vi "Convert numbers to Quadruped String.vi"(11 "Body Movements":T1) -> (3 "String to Write to Quadruped":string)   [LabVIEW 2014]
panel:
  out "String to Write to Quadruped 2":string
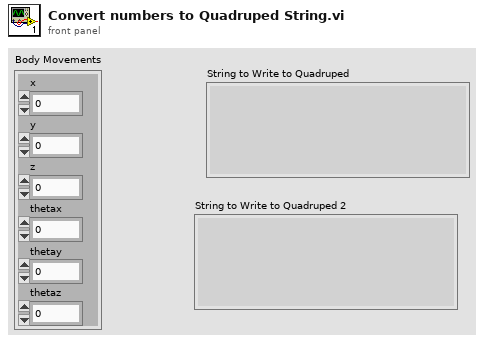
[diagram p1: front panel]
types:
  T1 = cluster{"x":sgl, "y":sgl, "z":sgl, "thetax":sgl, "thetay":sgl, "thetaz":sgl}
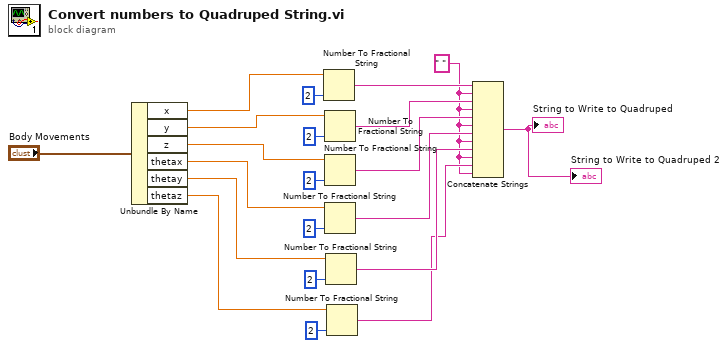
[diagram p0: block diagram]
diagram:
  w1 = " "
  n1 = Unbundle By Name("Body Movements") -> ("x"=w19:sgl, "y"=w17:sgl, "z"=w15:sgl, "thetax"=w13:sgl, "thetay"=w11:sgl, "thetaz"=w9:sgl)
  n2 = Number To Fractional String(number=w19, precision (6)=i16 2) -> (F-format string=w8:string)  [unwired: 2 in]
  n3 = Number To Fractional String(number=w17, precision (6)=i16 2) -> (F-format string=w7:string)  [unwired: 2 in]
  n4 = Number To Fractional String(number=w15, precision (6)=i16 2) -> (F-format string=w6:string)  [unwired: 2 in]
  n5 = Number To Fractional String(number=w13, precision (6)=i16 2) -> (F-format string=w5:string)  [unwired: 2 in]
  n6 = Number To Fractional String(number=w11, precision (6)=i16 2) -> (F-format string=w4:string)  [unwired: 2 in]
  n7 = Number To Fractional String(number=w9, precision (6)=i16 2) -> (F-format string=w3:string)  [unwired: 2 in]
  n8 = Concatenate Strings(w8, w1, w7, w1, w6, w1, w5, w1, w4, w1, w3, w1) -> (→"String to Write to Quadruped" →"String to Write to Quadruped 2":string)
